vi "SwerveGlobalData.vi"() -> ()   [LabVIEW 2016, in "Team900SwerveDrive.lvlib"]
uses:
  Team900SwerveDrive.lvlib
panel:
  in  "Write Coordinates":bool
  in  "Coordinates":cluster{"X":dbl, "Y":dbl, "Heading":dbl}={"X"=0.0, "Y"=0.0, "Heading"=90.0}
  in  "Drive Train Absolute Offsets (ticks)":dbl[](array[numeric])=[-0.395, 1.11, 1.68, -1.896]
  out "Wheel Angle Invert":bool
  in  "Wheel Speed TPI":dbl=2292.3908 format="%#_10g"
  in  "Drive Train Wheel Angles (rad)":cluster{"FL":dbl, "FR":dbl, "RL":dbl, "RR":dbl}={"FL"=-0.395, "FR"=1.11, "RL"=1.68, "RR"=-1.896}
  in  "Input Coordinates":cluster{"X":dbl, "Y":dbl, "Heading":dbl}={"X"=0.0, "Y"=0.0, "Heading"=90.0}
  in  "Absolute Encoder TPR":dbl=162.97466
  in  "Robot Width":dbl=24.5
  in  "Robot Length":dbl=24.5
  # "Static variables whose default\nvalues should be set here:"
  # "Variables which are set only\nin Begin.vi and read elsewhere:"
  # "Variables periodically written and read within code:"
  # "Setting these variables for each robot:\n\nValues for offsets should not be set here, but\nshould be set using SaveOffsets.vi or through \nthe webdash (as the code currently expects \noffsets in a .ini file in a flash drive on the \nroboRIO).\n\nValues for Robot Length/Width should be  \nmeasured in inches from center of wheel to\ncenter of wheel.\n\nAbsolute Encoder TPR (ticks per radian) is \ncurrently 1024/(2*pi), shouldn't need to be\nchanged.\n\nWheel Speed TPI (ticks per inch) should be \nchanged as necessary if something like \nwheel diameter or the gearing between the\nencoders and the wheels ever changes. This\ndoesn't really correspond to ticks on the \nencoder, but to values of sensor position as\noutput by the quadrature encoder (since quad\nencoders read each tick 4x)."
  # "(see LoadOffsets.vi\nor SaveOffsets.vi)"
  # "(see OpenSwerveDrive.vi)"
  # "This VI is mostly internal, but the user code\nwill need to set Coordinates itself within\nPeriodic Tasks.vi. When code from outside\nthis periodic tasks loop needs to set the \ncoordinates, it should set 'Input Coordinates,'\nthen set 'Write Coordinates' to True, as any\ndirect changes to 'Coordinates' outside of this\nloop may be accidentally overwritten.\n\nThought: In 2015RobotCode/Periodic Tasks.vi\nthere is a loop which handles these variables,\nas well as getting inputs for the navigation,\nzeroing/offsetting/inverting the yaw to be\nconsistent with the rest of the code, etc., and \nthis loop should be integrated into the \nswerve drive libraries as subVI's."
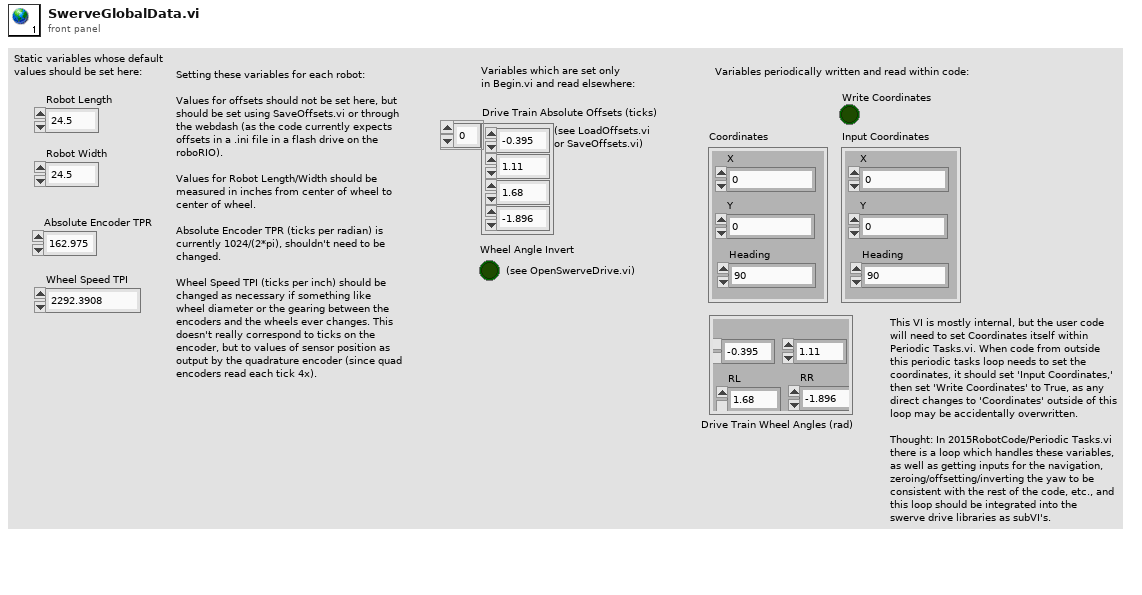
[diagram p1: front panel]
diagram:
